vi "Transform.vi"(7 "Type X":T1(ring), 8 "error in (no error)":errorcluster caption="entrée d'erreur (pas d'erreur)", 9 "y":string[][](array[string]), 10 "X":string[][](array[string]), 11 "MaxAbsScaler.lvclass":refnum<class "MaxAbsScaler.lvclass">) -> (0 "error in (no error)":errorcluster caption="entrée d'erreur (pas d'erreur)", 2 "Data":T2, 3 "MaxAbsScaler.lvclass":refnum<class "MaxAbsScaler.lvclass">)   [LabVIEW 2020, in "MaxAbsScaler.lvclass"]
doc: "Scale the data\n\nReturns : \n\n- X_new : ndarray array of shape (n_samples, n_features_new)\nTransformed array."
uses:
  MaxAbsScaler.lvclass
  MaxAbsScaler.lvclass/MaxAbsScaler.ctl
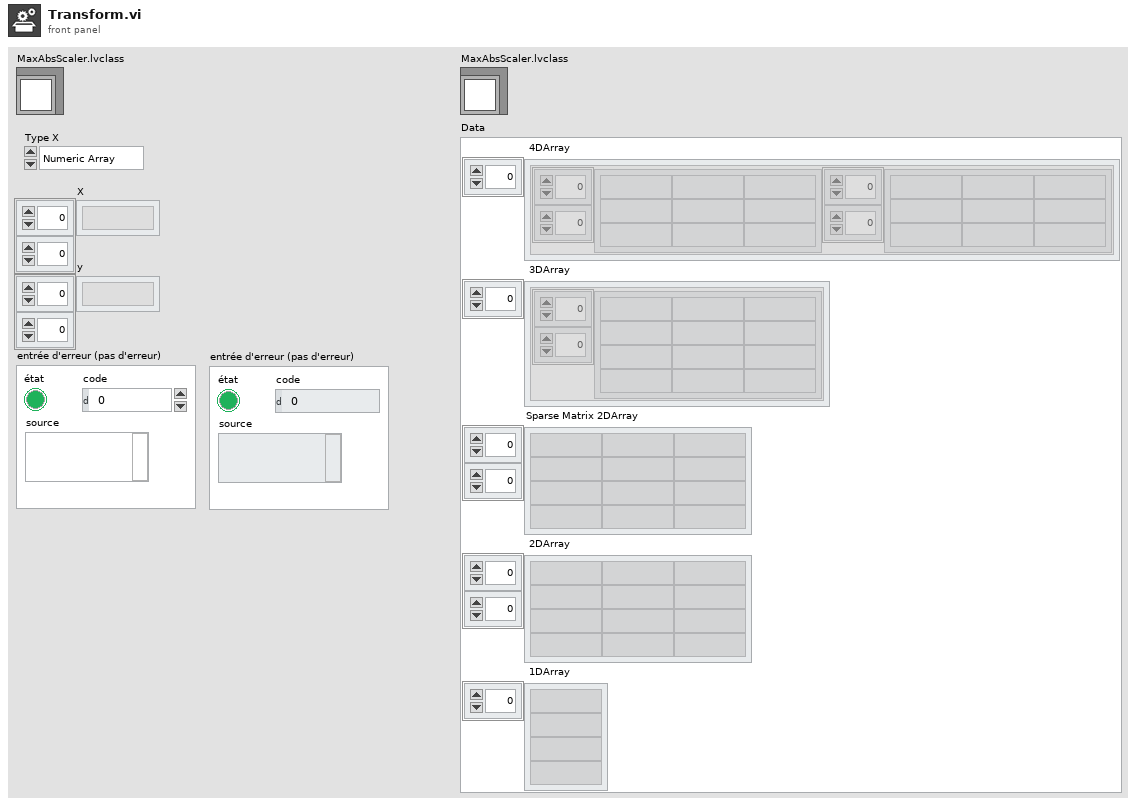
[diagram p1: front panel]
types:
  T1 = enum16{"Numeric Array", "String Array", "Sparse"}
  T2 = cluster{" 4DArray":cluster{"1":string[][], "2":string[][]}[], " 3DArray":cluster{"Tableau":string[][]}[], "Sparse Matrix 2DArray":string[][], " 2DArray":string[][], " 1DArray":string[]}
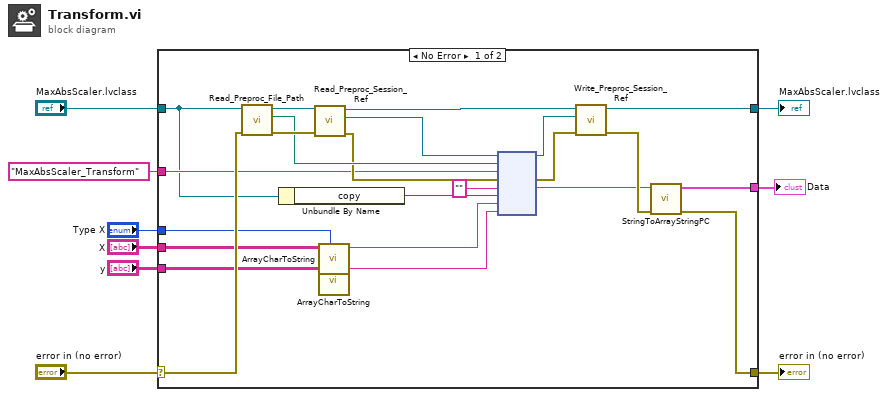
[diagram p0: block diagram]
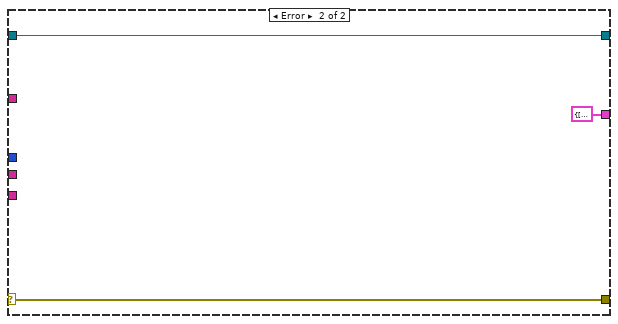
[diagram p2: hidden frame]
diagram:
  n1 = case shown="No Error" "error in (no error)" {
    selector: "error in (no error)" -> [w22 w35]
    tunnel: [w10 w35] -> w8
    tunnel: [w14 w34] -> w6
    tunnel: "MaxAbsScaler.lvclass" -> [w20 w34]
    tunnel: "MaxAbsScaler_Transform" ("Fonction") -> [w21 _]
    tunnel: [w11 T2 {" 4DArray"=[], " 3DArray"=[], "Sparse Matrix 2DArray"=[], " 2DArray"=[], " 1DArray"=[]} ("Data")] -> w4
    tunnel: "X" -> [w19 _]
    tunnel: "y" -> [w16 _]
    tunnel: "Type X" -> [w17 _]
    frame No Error {
      n2 = call-dynamic "Read_Preproc_File_Path.vi"("error in (no error)"=w22, "Python in"=w20) -> ("error out"=w31:errorcluster, "File_Path"=w28:path, "Python out"=w32:refnum<class "MaxAbsScaler.lvclass">)  [unwired: 7 in]
      n3 = Unbundle By Name(w20) -> ("copy"=w23:bool)
      n4 = call-dynamic "Read_Preproc_Session_Ref.vi"("error in (no error)"=w31, "Python in"=w32) -> ("error out"=w27:errorcluster, "Session_ref"=w29:refnum<k35>, "Python out"=w30:refnum<class "MaxAbsScaler.lvclass">)  [unwired: 7 in]
      n5 = call "ArrayCharToString.vi"("Type"=w17, "TAB"=w19) -> ("Instruction"=w18:string)  [unwired: 9 in]
      n6 = call "ArrayCharToString.vi"("TAB"=w16) -> ("Instruction"=w15:string)  [unwired: 10 in]
      n7 = node(w29, w28, w21, w27, "", w23, w18, w15) -> (w25:refnum<k35>, w26:errorcluster, w12:string)  [unwired: 3 in, 2 out]
      n8 = call-dynamic "Write_Preproc_Session_Ref.vi"("error in (no error)"=w26, "Session_ref"=w25, "Python in"=w30) -> ("error out"=w13:errorcluster, "Python out"=w14:refnum<class "MaxAbsScaler.lvclass">)  [unwired: 7 in]
      n9 = call "StringToArrayStringPC.vi"("sortie d'erreur"=w13, "Return value"=w12) -> ("sortie d'erreur"=w10:errorcluster, "Data"=w11:T2)  [unwired: 8 in]
    }
    frame Error {
    }
  }
  "error in (no error)" <- w8
  "MaxAbsScaler.lvclass" <- w6
  "Data" <- w4
